vi "Monitor.vi"(0 "host name":string="higgsino.physics.ucsb.edu", 1 "binding key":string[](array[string])=["#"], 2 "queue \nname":string="monitor", 3 "error (in)":errorcluster, 4 "exchange name":u16(ring) items=["requests", "alerts"]) -> (5 "error out":errorcluster)   [LabVIEW 2016]
uses:
  C:/Program Files (x86)/National Instruments/LabVIEW 2016/vi.lib/Distrio/LabbitMQ/RabbitMQ.Client.dll
  Program Files (x86)/National Instruments/LabVIEW 2016/vi.lib/Distrio/LabbitMQ/RabbitMQ.Client.dll
  <vilib>/Distrio/LabbitMQ/Queue/Queue.lvclass
  <vilib>/Distrio/LabbitMQ/Connection/Connection.lvclass
panel:
  in  "stop":bool
  in  "Tab Control":enum32{"AMQP Settings", "Logger"}(tab)
  out "Log":string
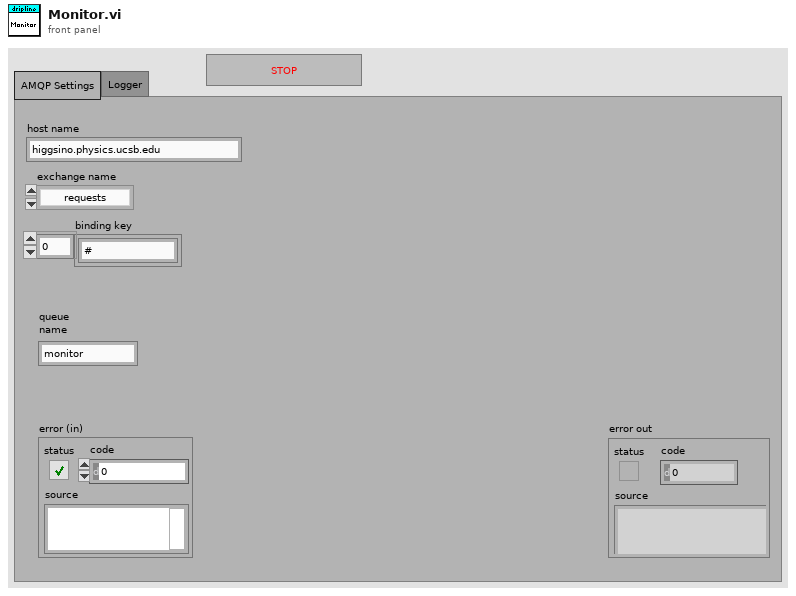
[diagram p1: front panel]
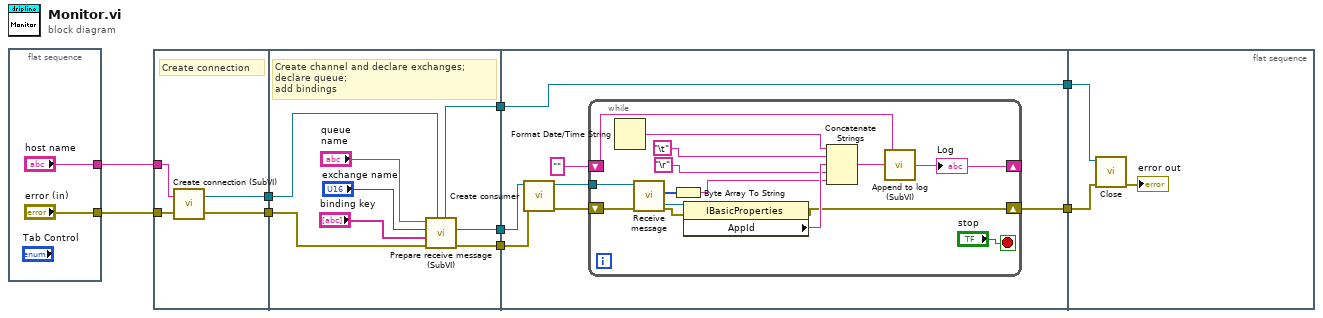
[diagram p0: block diagram]
diagram:
  n1 = flat-sequence {
    tunnel: ["error (in)"] -> w7
    tunnel: ["host name"] -> w6
    frame #0 {
    }
  }
  n2 = flat-sequence {
    tunnel: [w13] -> w9
    tunnel: [w12] -> w8
    tunnel: w6 -> [w15]
    tunnel: w7 -> [w14]
    tunnel: w9 -> [w18]
    tunnel: w8 -> [w17]
    tunnel: [w20] -> w4
    tunnel: [w19] -> w3
    tunnel: [w16] -> w1
    tunnel: [w29] -> w5
    tunnel: w4 -> [w26]
    tunnel: w3 -> [w25]
    tunnel: [w24] -> w2
    tunnel: w1 -> [w24]
    tunnel: w5 -> [w47]
    tunnel: w2 -> [w46]
    frame #0 {
      # "Create connection"
      n3 = call "Create connection (SubVI).vi"("error in (no error)"=w14, "host name"=w15) -> ("error out"=w12:errorcluster, "Connection out"=w13:refnum<class "Connection.lvclass">)
    }
    frame #1 {
      # "Create channel and declare exchanges; declare queue;\nadd bindings"
      n4 = call "Prepare receive message (SubVI).vi"("Connection in"=w18, "error in (no error)"=w17, "binding key"="binding key", "exchange name"="exchange name", "queue \nname"="queue \nname") -> ("error out"=w19:errorcluster, "Queue out"=w20:refnum<class "Queue.lvclass">, "Connection out"=w16:refnum<class "Connection.lvclass">)  [unwired: 2 out]
    }
    frame #2 {
      n5 = call <vilib>:"Create consumer.vi"("error in (no error)"=w25, "Queue in"=w26) -> ("error out"=w28:errorcluster, "Queue out"=w30:refnum<class "Queue.lvclass">)  [unwired: 8 in]
      n6 = while {
        tunnel: w30 -> [w45]
        shift-right: [w31] -> w29
        shift-left: w28 -> [w44]
        shift-right: [w40] -> _
        shift-left: "" -> [w41]
        stop <- "stop" stop-if-true
        n7 = Format Date/Time String() -> (date/time string=w38:string)  [unwired: 3 in]
        n8 = call <vilib>:"Receive message.vi"("error in (no error)"=w44, "Consumer in"=w45) -> ("error out"=w32:errorcluster, "message body"=w43:u8[], "MessageProperties"=w39:refnum<k24>)  [unwired: 4 in, 3 out]
        n9 = Byte Array To String(unsigned byte array=w43) -> (string=w34:string)
        n10 = property class="IBasicProperties"(reference=w39, error in=w32) -> (error out=w31:errorcluster, "AppId"=w36:string)  [unwired: 1 out]
        n11 = Concatenate Strings(w38, "\t", w36, "\r", w34) -> (w33:string)
        n12 = call "Append to log (SubVI).vi"("to append"=w33, "log in"=w41) -> ("log out"=w40:string)  [unwired: 1 in]
        "Log" <- w40
      }
    }
    frame #3 {
      n13 = call <vilib>:"Close.vi"("error in (no error)"=w47, "Connection in"=w46) -> ("error out"=→"error out":errorcluster)  [unwired: 8 in, 1 out]
    }
  }
